vi "Update MCP Server.vi"() -> ()   [LabVIEW 2025, in "Tools.lvlib"]
uses:
  Tools.lvlib
  Server Creator Data.ctl
  MCP Creator States.ctl
  PyServer/PyServer.lvclass
panel:
  in  "Server Name 2":string
  in  "Tab Control":enum32{"Configuration", "Python Code"}(tab)
  in  "Library Path":path
  in  "Remove Tool":bool
  in  "Description":string
  in  "Tools":i32[](listbox)
  in  "Server Name":string
  in  "Add_Tool":bool
  in  "Add Folder":bool
  out "Python String":string
  in  "error in (no error)":errorcluster
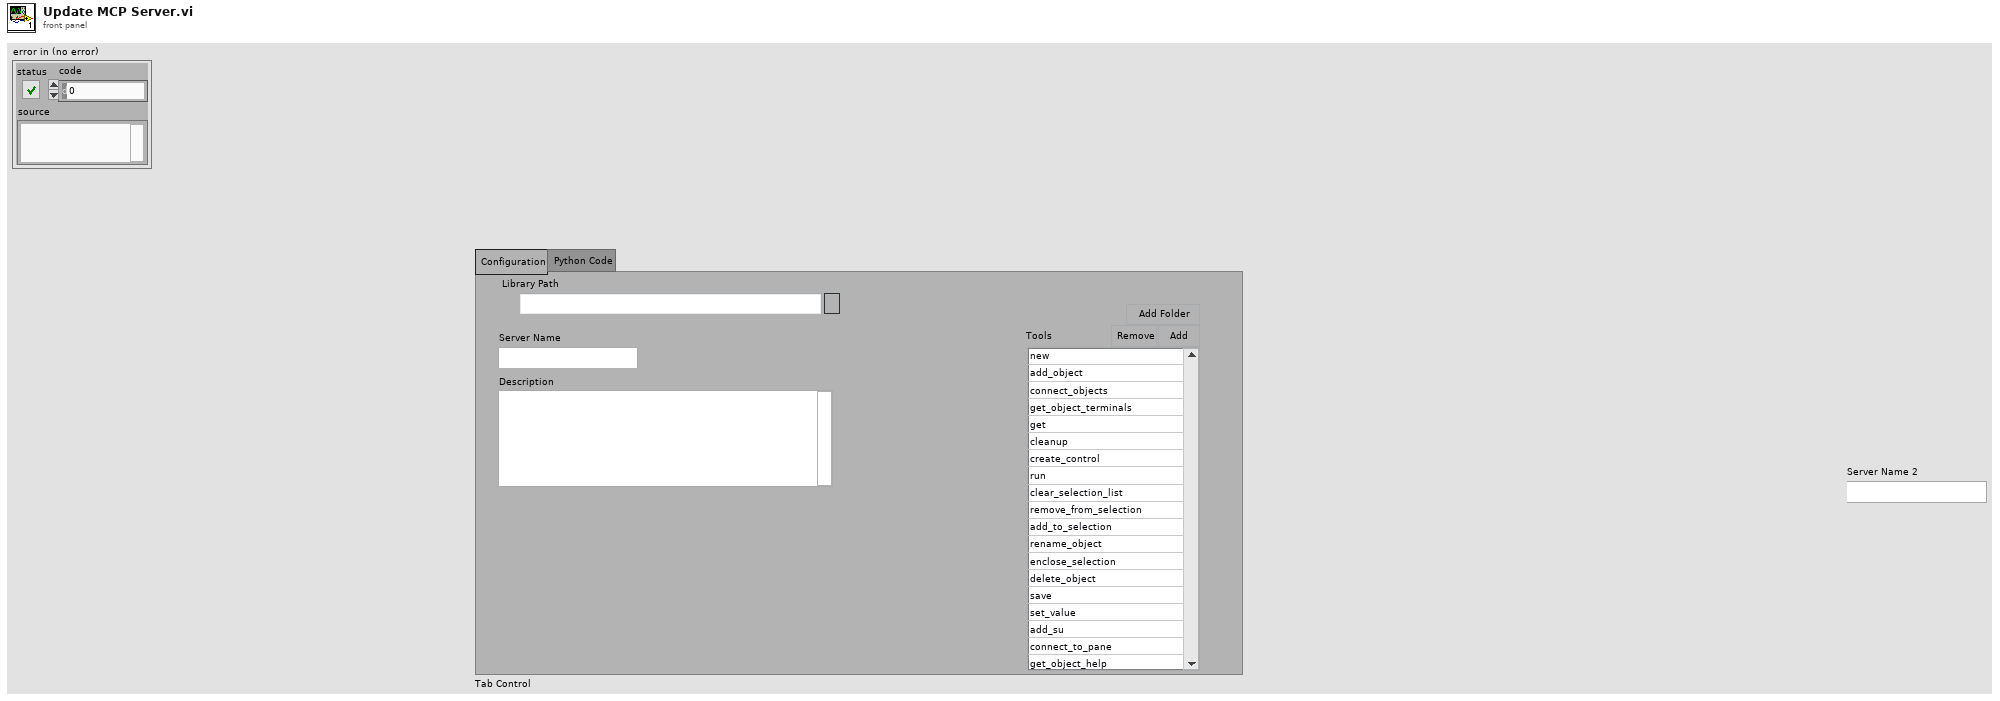
[diagram p1: front panel]
types:
  T1 = typedef "Tools.lvlib/MCP Creator States.ctl" = enum16{"Wait For Event", "Update UI", "Update Server", "Load Project"}
  T2 = typedef "Tools.lvlib/Server Creator Data.ctl" = cluster{"Name":string, "Description":string, "Tools":path[], "Project Path":path}
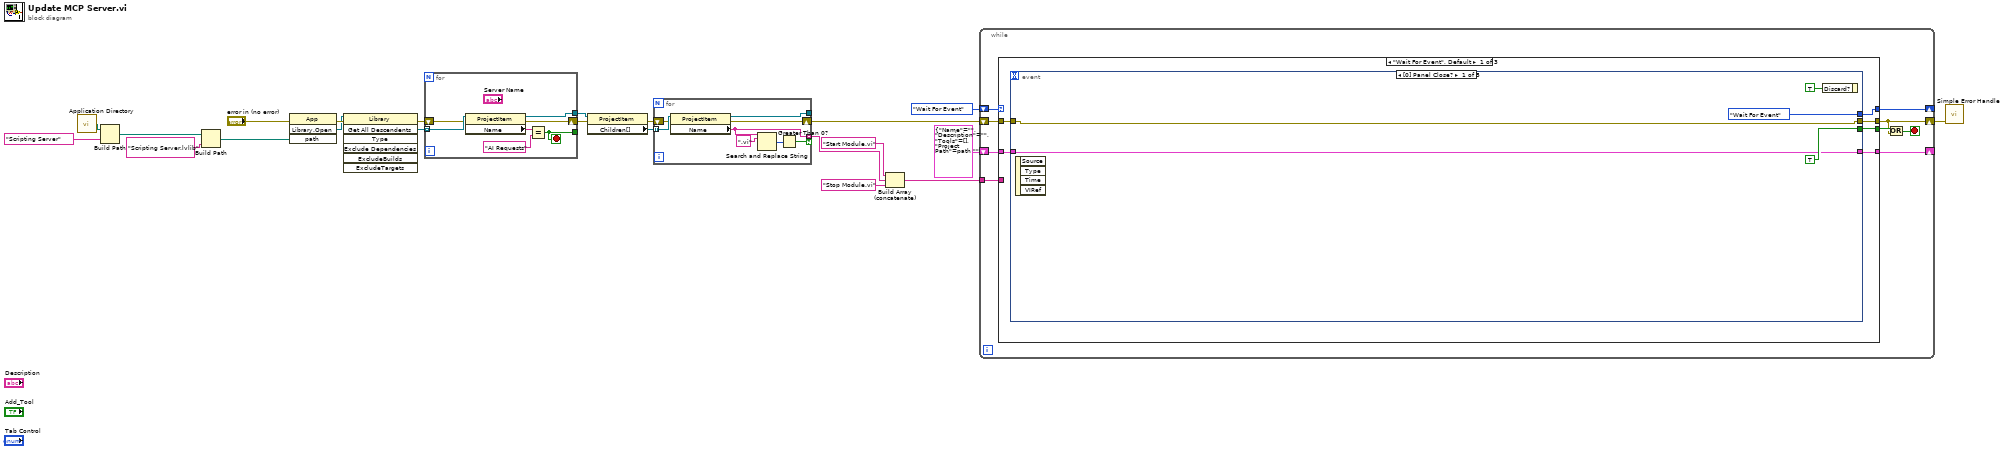
[diagram p0: block diagram]
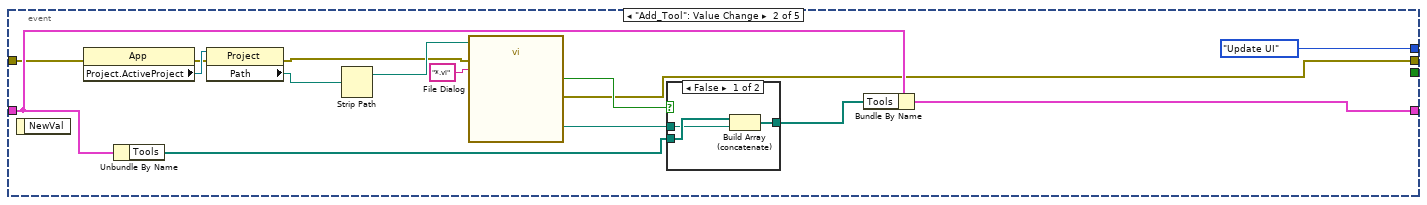
[diagram p2: hidden frame]
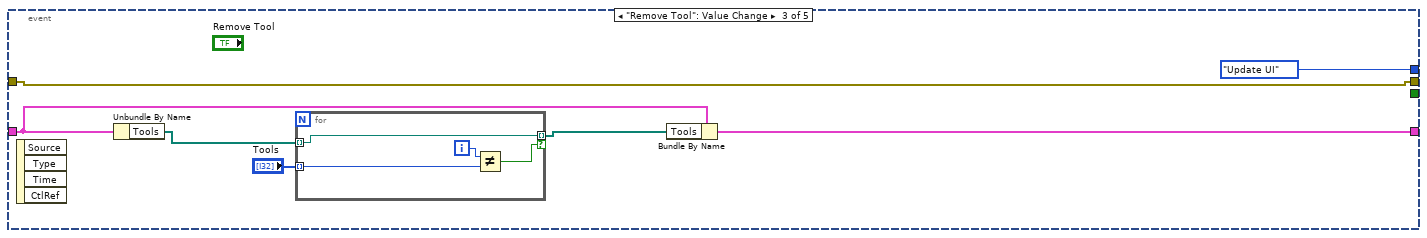
[diagram p4: hidden frame]
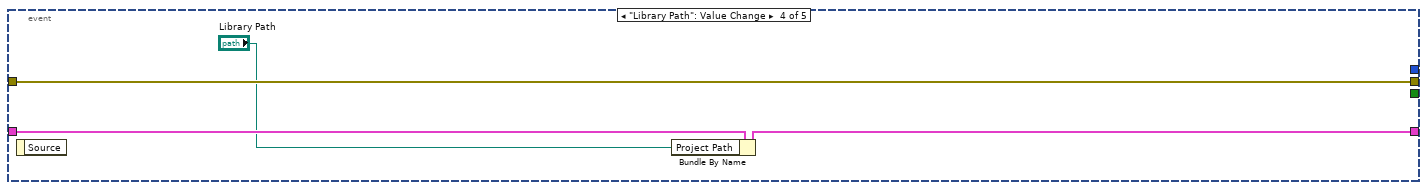
[diagram p5: hidden frame]
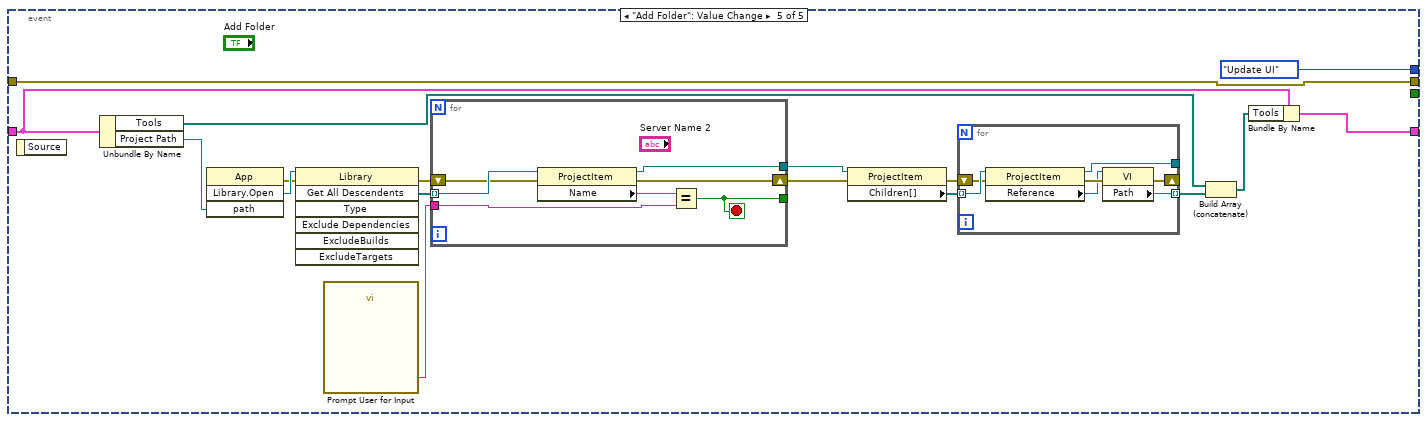
[diagram p6: hidden frame]
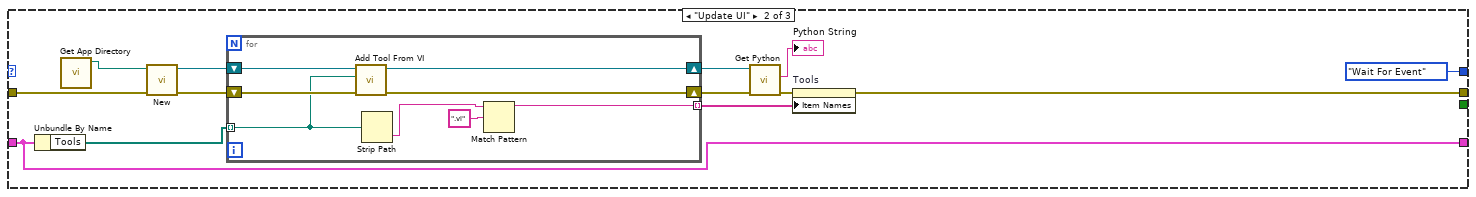
[diagram p7: hidden frame]
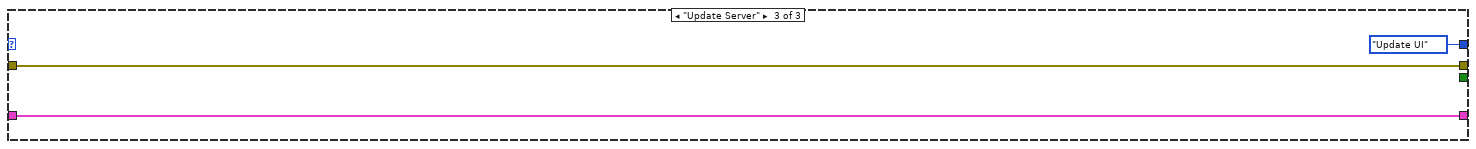
[diagram p8: hidden frame]
diagram:
  n1 = call <vilib>:"Application Directory.vi"() -> ("Application Directory"=w13:path)
  n2 = Build Path(base path=w13, name or relative path="Scripting Server" ("format string")) -> (appended path=w11:path)
  n3 = Build Path(base path=w11, name or relative path="Scripting Server.lvlib" ("format string")) -> (appended path=w9:path)
  n4 = invoke class="App" method="Library.Open"(error in="error in (no error)", "path"=w9) -> (error out=w8:errorcluster, "Open Library"=w7:refnum<vi>)  [unwired: 2 in, 2 out]
  n5 = invoke class="Library" method="Get All Descendents"(reference=w7, error in=w8) -> (error out=w16:errorcluster, "All Descendents"=w17:refnum<vi>[])  [unwired: 5 in, 5 out]
  n6 = for {
    tunnel: w17 -> [w29] mode=indexing
    tunnel: [w28] -> w15
    shift-right: [w24] -> w14
    shift-left: w16 -> [w25]
    tunnel: [w23] -> _
    stop <- w23 stop-if-true
    n7 = property class="ProjectItem"(reference=w29, error in=w25) -> (reference out=w28:refnum<vi>, error out=w24:errorcluster, "Name"=w27:string)
    n8 = Equal?(x=w27, y="AI Requests") -> (x = y?=w23:bool)
  }
  n9 = property class="ProjectItem"(reference=w15, error in=w14) -> (error out=w21:errorcluster, "Children[]"=w22:refnum<vi>[])  [unwired: 1 out]
  n10 = for {
    tunnel: w22 -> [w37] mode=indexing
    tunnel: [w36] -> _
    tunnel: [w33] -> w20 mode=indexing if=w30
    shift-right: [w34] -> w4
    shift-left: w21 -> [w35]
    n11 = property class="ProjectItem"(reference=w37, error in=w35) -> (reference out=w36:refnum<vi>, error out=w34:errorcluster, "Name"=w33:string)
    n12 = Search and Replace String(input string=w33, search string=".vi" ("regular expression")) -> (number of replacements=w31:i32)  [unwired: 6 in, 3 out]
    n13 = Greater Than 0?(x=w31) -> (x > 0?=w30:bool)
  }
  n14 = Build Array (concatenate)("Start Module.vi" ("y"), w20, "Stop Module.vi" ("y")) -> (w2:string[])
  n15 = while {
    shift-right: [w46] -> _
    shift-left: T2 {"Name"="", "Description"="", "Tools"=[], "Project Path"=path ""} -> [w45]
    shift-right: [w41] -> w1
    shift-left: w4 -> [w44]
    shift-right: [w39] -> _
    shift-left: MCP_Creator_States."Wait For Event" -> [w40]
    tunnel: w2 -> [w38]
    stop <- w42 stop-if-true
    n16 = case shown="\"Wait For Event\", Default" w40 {
      tunnel: [w52 w127 w146] -> w46
      tunnel: w45 -> [w51 w127 w146]
      tunnel: w44 -> [w50 w128 w145]
      tunnel: [w49 _ _] -> w43
      tunnel: [w48 w123 w145] -> w41
      tunnel: [w47 MCP_Creator_States."Wait For Event" MCP_Creator_States."Update UI"] -> w39
      tunnel: w38 -> [_ _ _]
      frame "Wait For Event", Default {
        n17 = event shown="[0] Panel Close?" {
          selector: _ -> [_ _ _ _ _]
          dyn-events: _ -> [_ _ _ _ _]
          timeout: _ -> [_ _ _ _ _]
          tunnel: [TRUE ("Discard?") _ _ _ _] -> w49
          tunnel: [w54 w72 w81 w89 w96] -> w52
          tunnel: w51 -> [w54 w71 w80 w91 w107]
          tunnel: w50 -> [w55 w62 w83 w90 w108]
          tunnel: [w55 w59 w83 w90 w108] -> w48
          tunnel: [MCP_Creator_States."Wait For Event" MCP_Creator_States."Update UI" MCP_Creator_States."Update UI" _ MCP_Creator_States."Update UI"] -> w47
          event Panel Close? {
            n18 = event-data() -> ()  [unwired: 1 in, 4 out]
            n19 = event-data("Discard?"=TRUE) -> ()  [unwired: 1 in, 1 out]
          }
          event "Add_Tool": Value Change {
            n20 = event-data() -> ()  [unwired: 1 in, 1 out]
            n21 = property class="App"(error in=w62) -> (error out=w61:errorcluster, "Project.ActiveProject"=w67:refnum<vi>)  [unwired: 1 in, 1 out]
            n22 = Unbundle By Name(w71) -> ("Tools"=w70:path[])
            n23 = property class="Project"(reference=w67, error in=w61) -> (error out=w60:errorcluster, "Path"=w66:path)  [unwired: 1 out]
            n24 = Strip Path(path=w66) -> (stripped path=w65:path)  [unwired: 1 out]
            n25 = call "File Dialog"("start path"=w65, "error in"=w60, "pattern (all files)"="*.vi" ("pattern label")) -> ("selected path"=w64:path, "cancelled"=w63:bool, "error out"=w59:errorcluster)  [unwired: 9 in, 1 out]
            n26 = case shown="False" w63 {
              tunnel: w70 -> [w75 w76]
              tunnel: [w74 w76] -> w69
              tunnel: w64 -> [w73 _]
              frame False {
                n27 = Build Array (concatenate)(w75, w73) -> (w74:path[])
              }
              frame True {
              }
            }
            n28 = Bundle By Name(cluster=w71, "Tools"=w69) -> (w72:T2)
          }
          event "Remove Tool": Value Change {
            n29 = event-data() -> ()  [unwired: 1 in, 4 out]
            n30 = Unbundle By Name(w80) -> ("Tools"=w79:path[])
            n31 = for {
              tunnel: w79 -> [w85] mode=indexing
              tunnel: "Tools" -> [w86] mode=indexing
              tunnel: [w85] -> w77 mode=indexing if=w84
              i -> [w87]
              n32 = Not Equal?(x=w87, y=w86) -> (x != y?=w84:bool)
            }
            n33 = Bundle By Name(cluster=w80, "Tools"=w77) -> (w81:T2)
          }
          event "Library Path": Value Change {
            n34 = event-data() -> ()  [unwired: 1 in, 1 out]
            n35 = Bundle By Name(cluster=w91, "Project Path"="Library Path") -> (w89:T2)
          }
          event "Add Folder": Value Change {
            n36 = event-data() -> ()  [unwired: 1 in, 1 out]
            n37 = Unbundle By Name(w107) -> ("Tools"=w95:path[], "Project Path"=w98:path)
            n38 = invoke class="App" method="Library.Open"("path"=w98) -> (error out=w105:errorcluster, "Open Library"=w106:refnum<vi>)  [unwired: 3 in, 2 out]
            n39 = invoke class="Library" method="Get All Descendents"(reference=w106, error in=w105) -> (error out=w102:errorcluster, "All Descendents"=w101:refnum<vi>[])  [unwired: 5 in, 5 out]
            n40 = call "Prompt User for Input"() -> ("Folder Name"=w97:string)  [unwired: 17 in, 2 out]
            n41 = for {
              tunnel: w101 -> [w115] mode=indexing
              tunnel: [w114] -> w103
              shift-right: [w111] -> w104
              shift-left: w102 -> [w112]
              tunnel: [w110] -> _
              tunnel: w97 -> [w109]
              stop <- w110 stop-if-true
              n42 = property class="ProjectItem"(reference=w115, error in=w112) -> (reference out=w114:refnum<vi>, error out=w111:errorcluster, "Name"=w113:string)
              n43 = Equal?(x=w113, y=w109) -> (x = y?=w110:bool)
            }
            n44 = property class="ProjectItem"(reference=w103, error in=w104) -> (error out=w100:errorcluster, "Children[]"=w99:refnum<vi>[])  [unwired: 1 out]
            n45 = for {
              tunnel: w99 -> [w122] mode=indexing
              tunnel: [w121] -> _
              shift-right: [w118] -> _
              shift-left: w100 -> [w120]
              tunnel: [w116] -> w93 mode=indexing
              n46 = property class="ProjectItem"(reference=w122, error in=w120) -> (reference out=w121:refnum<vi>, error out=w119:errorcluster, "Reference"=w117:refnum<vi>)
              n47 = property class="VI"(reference=w117, error in=w119) -> (error out=w118:errorcluster, "Path"=w116:path)  [unwired: 1 out]
            }
            n48 = Build Array (concatenate)(w95, w93) -> (w94:path[])
            n49 = Bundle By Name(cluster=w107, "Tools"=w94) -> (w96:T2)
          }
        }
      }
      frame "Update UI" {
        n50 = Unbundle By Name(w127) -> ("Tools"=w126:path[])
        n51 = call "Get App Directory.vi"() -> ("appended path"=w130:path)  [unwired: 11 in]
        n52 = call "New.vi"("error in (no error)"=w128, "Server Path"=w130) -> ("error out"=w133:errorcluster, "PyServer out"=w131:refnum<class "PyServer.lvclass">)  [unwired: 8 in]
        n53 = for {
          tunnel: w126 -> [w139] mode=indexing
          shift-right: [w142] -> w129
          shift-left: w133 -> [w143]
          shift-right: [w140] -> w132
          shift-left: w131 -> [w141]
          tunnel: [w136] -> w125 mode=indexing
          n54 = call "Add Tool From VI.vi"("error in (no error)"=w143, "vi path"=w139, "PyServer in"=w141) -> ("error out"=w142:errorcluster, "PyServer out"=w140:refnum<class "PyServer.lvclass">)  [unwired: 7 in]
          n55 = Strip Path(path=w139) -> (name=w138:string)  [unwired: 1 out]
          n56 = Match Pattern(string=w138, regular expression=".vi") -> (before substring=w136:string)  [unwired: 1 in, 3 out]
        }
        n57 = call "Get Python.vi"("error in (no error)"=w129, "PyServer in"=w132) -> ("error out"=w124:errorcluster, "resulting string"=→"Python String":string)  [unwired: 7 in, 1 out]
        n58 = property on="Tools" class="LstBox (strict)"(error in=w124, "Item Names"=w125) -> (error out=w123:errorcluster)  [unwired: 1 in, 1 out]
      }
      frame "Update Server" {
      }
    }
    n59 = Or(x=w43, y=w41) -> (x .or. y?=w42:bool)
  }
  n60 = call <vilib>:"Simple Error Handler.vi"("error in (no error)"=w1) -> ()  [unwired: 4 in, 5 out]
